vi "PIM Calculate Fim Range.vi"(5 "Custom Sweep":T1 {"Stop 2" format="%.2f"; "Start 2" format="%.2f"; "Stop 1" format="%.2f"; "Start 1" format="%.2f"}, 7 "Base Order (0)":u8, 8 "Low order IM? (T)":bool=TRUE) -> (1 "Fim, high":dbl, 2 "Fim, low":dbl)   [LabVIEW 2011]
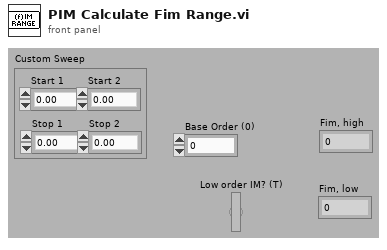
[diagram p1: front panel]
types:
  T1 = cluster{"Start 1":dbl, "Stop 1":dbl, "Start 2":dbl, "Stop 2":dbl}
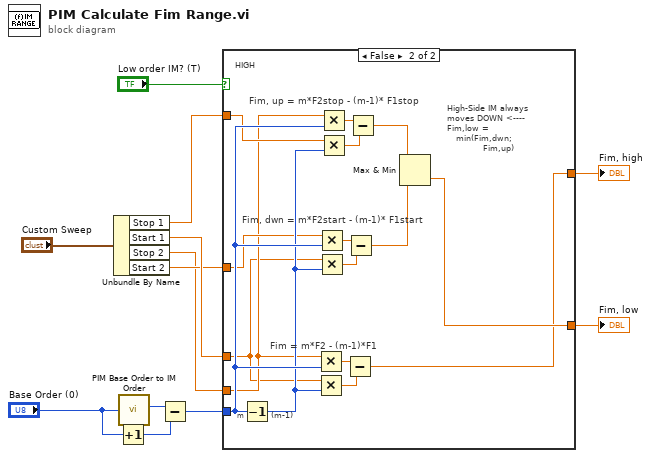
[diagram p0: block diagram]
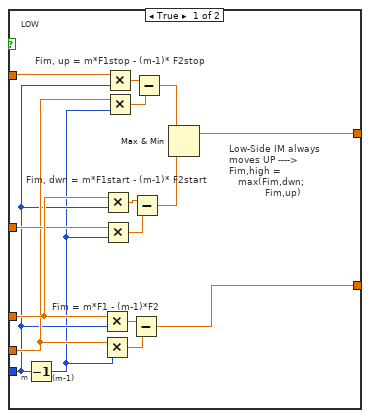
[diagram p2: hidden frame]
diagram:
  n1 = Unbundle By Name("Custom Sweep") -> ("Stop 1"=w7:dbl, "Start 1"=w9:dbl, "Stop 2"=w6:dbl, "Start 2"=w8:dbl)
  n2 = Increment(x="Base Order (0)") -> (x+1=w11:u8)
  n3 = call "PIM Base Order to IM Order.vi"("Base Order (0)"="Base Order (0)") -> ("IM Order"=w12:u8)  [unwired: 5 out]
  n4 = Subtract(x=w12, y=w11) -> (x-y=w5:u8)
  n5 = case shown="False" "Low order IM? (T)" {
    tunnel: w9 -> [w24 w33]
    tunnel: w8 -> [w23 w35]
    tunnel: w7 -> [w22 w36]
    tunnel: w6 -> [w21 w34]
    tunnel: w5 -> [w20 w40]
    tunnel: [w14 w31] -> w3
    tunnel: [w13 w32] -> w2
    frame True {
      # "Low-Side IM always\nmoves UP ---->\nFim,high = \n   max(Fim,dwn;\n            Fim,up)"
      # "(m-1)"
      # "m"
      # "LOW"
      # "Fim, up = m*F1stop - (m-1)* F2stop"
      # "Fim, dwn = m*F1start - (m-1)* F2start"
      # "Fim = m*F1 - (m-1)*F2"
      n6 = Decrement(x=w20) -> (x-1=w17:u8)
      n7 = Multiply(x=w24, y=w20) -> (x*y=w28:dbl)
      n8 = Multiply(x=w21, y=w17) -> (x*y=w27:dbl)
      n9 = Multiply(x=w24, y=w20) -> (x*y=w25:dbl)
      n10 = Multiply(x=w23, y=w17) -> (x*y=w26:dbl)
      n11 = Multiply(x=w22, y=w20) -> (x*y=w19:dbl)
      n12 = Multiply(x=w21, y=w17) -> (x*y=w18:dbl)
      n13 = Subtract(x=w28, y=w27) -> (x-y=w13:dbl)
      n14 = Subtract(x=w25, y=w26) -> (x-y=w15:dbl)
      n15 = Subtract(x=w19, y=w18) -> (x-y=w16:dbl)
      n16 = Max & Min(x=w16, y=w15) -> (max(x,y)=w14:dbl)  [unwired: 1 out]
    }
    frame False {
      # "High-Side IM always\nmoves DOWN <----\nFim,low = \n   min(Fim,dwn;\n            Fim,up)"
      # "m"
      # "(m-1)"
      # "HIGH"
      # "Fim, up = m*F2stop - (m-1)* F1stop"
      # "Fim, dwn = m*F2start - (m-1)* F1start"
      # "Fim = m*F2 - (m-1)*F1"
      n17 = Decrement(x=w40) -> (x-1=w37:u8)
      n18 = Multiply(x=w34, y=w40) -> (x*y=w44:dbl)
      n19 = Multiply(x=w33, y=w37) -> (x*y=w43:dbl)
      n20 = Multiply(x=w35, y=w40) -> (x*y=w41:dbl)
      n21 = Multiply(x=w33, y=w37) -> (x*y=w42:dbl)
      n22 = Multiply(x=w34, y=w40) -> (x*y=w39:dbl)
      n23 = Multiply(x=w36, y=w37) -> (x*y=w38:dbl)
      n24 = Subtract(x=w44, y=w43) -> (x-y=w31:dbl)
      n25 = Subtract(x=w41, y=w42) -> (x-y=w29:dbl)
      n26 = Subtract(x=w39, y=w38) -> (x-y=w30:dbl)
      n27 = Max & Min(x=w30, y=w29) -> (min(x,y)=w32:dbl)  [unwired: 1 out]
    }
  }
  "Fim, low" <- w2
  "Fim, high" <- w3
